vi "Retrieve Selected Montage.vi"(11 "ListBox in":refnum<vi>) -> (2 "Value":i32, 3 "EEG Channels":T1(array[cluster]))   [LabVIEW 2016, in "Settings Editor.lvlib"]
uses:
  Settings Editor.lvlib
  CML Shared/EEG Channel Settings.ctl
  <vilib>/Utility/xml.llb/Read From XML File(string).vi
  CML Shared/CML Shared.lvlib
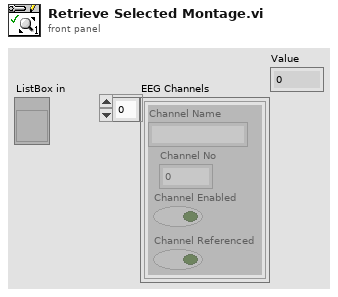
[diagram p1: front panel]
types:
  T1 = cluster{"Channel Name":string, "Channel No":u8, "Channel Enabled":bool, "Channel Referenced":bool}[]
  T2 = typedef "CML Shared.lvlib/EEG Channel Settings.ctl" = cluster{"16 EEG Channels":cluster{"Channel Name":string, "Channel No":u8, "Channel Enabled":bool, "Channel Referenced":bool}[], "Gain":u8}
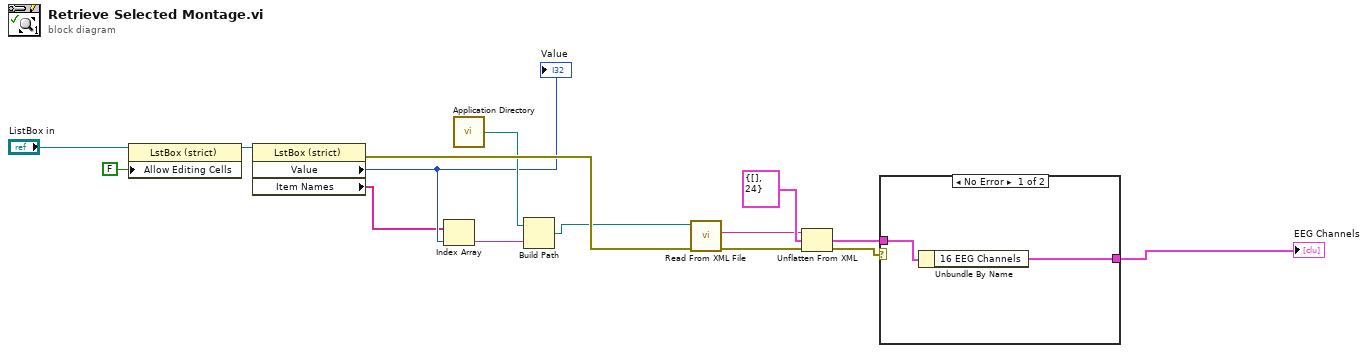
[diagram p0: block diagram]
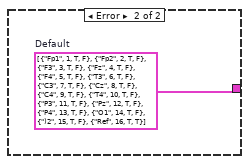
[diagram p2: hidden frame]
diagram:
  n1 = property class="LstBox (strict)"(reference="ListBox in", "Allow Editing Cells"=FALSE) -> (reference out=w3:refnum<vi>)  [unwired: 1 in, 1 out]
  n2 = property class="LstBox (strict)"(reference=w3) -> (error out=w11:errorcluster, "Value"=w5:i32, "Item Names"=w4:string[])  [unwired: 1 in, 1 out]
  "Value" <- w5
  n3 = Index Array(array=w4, index=w5) -> (element=w6:string)
  n4 = call <vilib>:"Application Directory.vi"() -> ("Application Directory"=w7:path)
  n5 = Build Path(base path=w7, name or relative path=w6) -> (appended path=w10:path)
  n6 = call-poly <vilib>:"Read From XML File.vi"("error in (no error)"=w11, "XML File Path"=w10) -> ("error out"=w9:errorcluster, "XML Elements"=w8:string)  [unwired: 7 in, 1 out]
  n7 = Unflatten From XML(xml string=w8, type=T2 {"16 EEG Channels"=[], "Gain"=24} ("EEG Channels"), error in (no error)=w9) -> (value=w13:T2, error out=w15:errorcluster)
  n8 = case shown="No Error" w15 {
    tunnel: w13 -> [w17 _]
    tunnel: [w16 w18] -> w14
    frame No Error {
      n9 = Unbundle By Name(w17) -> ("16 EEG Channels"=w16:T1)
    }
    frame Error {
      w18 = T1 [{"Channel Name"="Fp1", "Channel No"=1, "Channel Enabled"=TRUE, "Channel Referenced"=FALSE}, {"Channel Name"="Fp2", "Channel No"=2, "Channel Enabled"=TRUE, "Channel Referenced"=FALSE}, {"Channel Name"="F3", "Channel No"=3, "Channel Enabled"=TRUE, "Channel Referenced"=FALSE}, {"Channel Name"="Fz", "Channel No"=4, "Channel Enabled"=TRUE, "Channel Referenced"=FALSE}, {"Channel Name"="F4", "Channel No"=5, "Channel Enabled"=TRUE, "Channel Referenced"=FALSE}, {"Channel Name"="T3", "Channel No"=6, "Channel Enabled"=TRUE, "Channel Referenced"=FALSE}, {"Channel Name"="C3", "Channel No"=7, "Channel Enabled"=TRUE, "Channel Referenced"=FALSE}, {"Channel Name"="Cz", "Channel No"=8, "Channel Enabled"=TRUE, "Channel Referenced"=FALSE}, {"Channel Name"="C4", "Channel No"=9, "Channel Enabled"=TRUE, "Channel Referenced"=FALSE}, {"Channel Name"="T4", "Channel No"=10, "Channel Enabled"=TRUE, "Channel Referenced"=FALSE}, {"Channel Name"="P3", "Channel No"=11, "Channel Enabled"=TRUE, "Channel Referenced"=FALSE}, {"Channel Name"="Pz", "Channel No"=12, "Channel Enabled"=TRUE, "Channel Referenced"=FALSE}, {"Channel Name"="P4", "Channel No"=13, "Channel Enabled"=TRUE, "Channel Referenced"=FALSE}, {"Channel Name"="O1", "Channel No"=14, "Channel Enabled"=TRUE, "Channel Referenced"=FALSE}, {"Channel Name"=")2", "Channel No"=15, "Channel Enabled"=TRUE, "Channel Referenced"=FALSE}, {"Channel Name"="Ref", "Channel No"=16, "Channel Enabled"=TRUE, "Channel Referenced"=TRUE}]  # Default
    }
  }
  "EEG Channels" <- w14
